vi "CCE RRMA P03 SubVI092.vi"(11 "MOMENTOS INVARIANTES DE HU":dbl[](array[numeric])=[0.9997525383124077, 0.022047103684425993, 0.00047771658598479535, 0.0029255984598577215, 8.143259107920102e-07, 4.0976510303173995e-06, -2.948715981189433e-07]) -> (0 "logical OR":bool, 2 "min value":dbl, 3 "element":string)   [LabVIEW 2020]
doc: "Ceballos Conde Emanuel Rodríguez Ramírez Miguel Ángel 4MV6 Sistemas de visión artificial 2022/1\nEste vi contiene el funcionamiento de una neurona compet y a su vez la memoria que esta requiere para operar, este vi da como resultado el nombre del objeto en memoria que detecte la neurona respecto a la entrada"
panel:
  # "Ceballos Conde Emanuel\nRodríguez Ramírez Miguel Ángel\n4MV6\nSistemas de visión artificial\n2022/1"
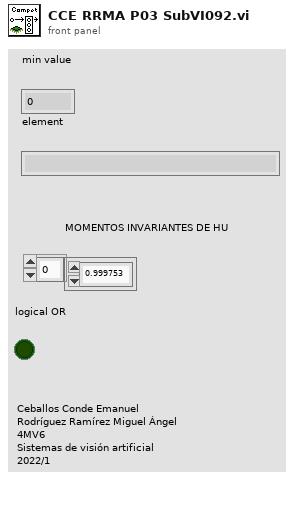
[diagram p1: front panel]
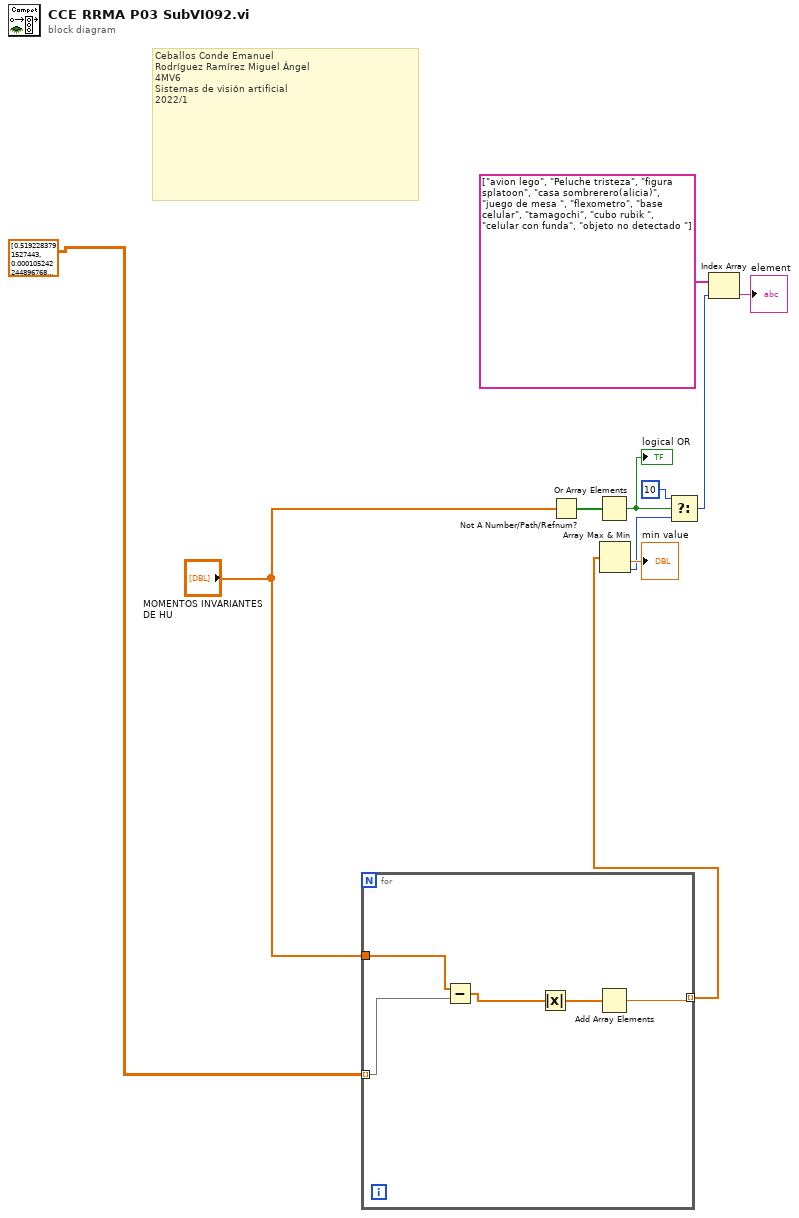
[diagram p0: block diagram]
diagram:
  # "Ceballos Conde Emanuel\nRodríguez Ramírez Miguel Ángel\n4MV6\nSistemas de visión artificial\n2022/1"
  n1 = for {
    tunnel: dbl[][] [[0.5192283791527443, 0.00010524224489676868, 0.00023093503031878737, 0.002747116953111497, -2.163434899542428e-06, -1.631754875336728e-07, -3.2739420591829756e-07], [0.21095107661760326, 0.01595986271622447, 4.949400639043596e-05, 1.1978617277908961e-05, 2.8346688754203954e-10, 1.6398931301230153e-08, -6.867159624347087e-11], [0.4288887655964658, 0.009415454186352368, 0.012033420327790544, 0.02011826479586343, 0.00026176116158367553, 0.0006671420323103025, 0.00017165759867374776], [0.7102944335284449, 0.1279529404783077, 0.022394775587162765, 0.031291183476929406, 0.0007857731665151314, 0.0005880056775055468, 0.00026210769195177824], [0.29417963302945593, 0.004165515842615368, 0.0015390598603548591, 0.0012929563727715582, 1.7987113084072917e-06, 2.074733938580927e-06, 3.021386057513566e-07], [0.46673797225998326, 0.046148731633019136, 0.007846861812457234, 0.0001557935635393273, 1.5532644585719549e-07, 5.379736285325735e-06, 7.44683778680196e-08], [0.29260614255709594, 0.002090369615318848, 0.0011947628157441528, 2.095431215326079e-05, -9.310360700685417e-10, -2.7608418594347163e-07, 3.18210776251984e-09], [1.795186281154134, 0.8056316642135564, 2.5256802378309153, 3.2624793312608937, -0.1865729966245102, 8.94674346139284, 9.363207213763449], [0.2577663021051355, 0.0036465611985897414, 8.823528777870509e-05, 0.0006426752115160472, 9.162468794514958e-08, -2.6178283817218796e-08, -1.225827794598232e-07], [0.9940282499120748, 0.0008256620447861698, 0.0016072838496001417, 0.014098497594470386, -1.106971441838275e-05, -2.616236971538891e-05, -6.619360363234656e-05]] ("MOMENTOS INVARIANTES DE HU") -> [w15] mode=indexing
    tunnel: "MOMENTOS INVARIANTES DE HU" -> [w16]
    tunnel: [w12] -> w2 mode=indexing
    n2 = Subtract(x=w16, y=w15) -> (x-y=w14:dbl[])
    n3 = Absolute Value(x=w14) -> (abs(x)=w13:dbl[])
    n4 = Add Array Elements(numeric array=w13) -> (sum=w12:dbl)
  }
  n5 = Not A Number/Path/Refnum?(number/path/refnum="MOMENTOS INVARIANTES DE HU") -> (NaN/Path/Refnum?=w7:bool[])
  n6 = Or Array Elements(Boolean array=w7) -> (logical OR=w8:bool)
  "logical OR" <- w8
  n7 = Array Max & Min(array=w2) -> (min value=→"min value":dbl, min index (indices)=w5:i32)  [unwired: 2 out]
  n8 = Select(t=10, s=w8, f=w5) -> (s? t:f=w6:i32)
  n9 = Index Array(array=string[] ["avion lego", "Peluche tristeza", "figura splatoon", "casa sombrerero(alicia)", "juego de mesa ", "flexometro", "base celular", "tamagochi", "cubo rubik ", "celular con funda", "objeto no detectado "], index=w6) -> (element=→"element":string)
